vi "Uniform Partially Matched Crossover(UPMX).vi"(9 "indpb":dbl=0.5 format="%#_13g", 10 "Ind 2":T1, 11 "Ind 1":T1) -> (2 "Child 2":T1, 3 "Child 1":T1)   [LabVIEW 2013, in "GA.lvclass"]
uses:
  GA.lvclass
  Controls/Solution_GA.ctl
panel:
  out "Child2 Schedule":u16[](array[numeric])
  out "Child 1 Schedule":u16[](array[numeric])
  out "p2":i32[](array[numeric])
  out "p1":i32[](array[numeric])
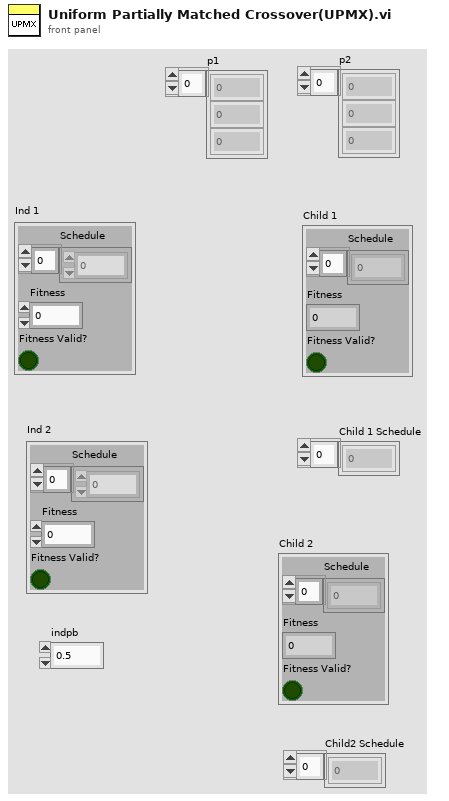
[diagram p1: front panel]
types:
  T1 = typedef "Solution_GA.ctl" = cluster{"Schedule":u16[], "Fitness":u16, "Fitness Valid?":bool}
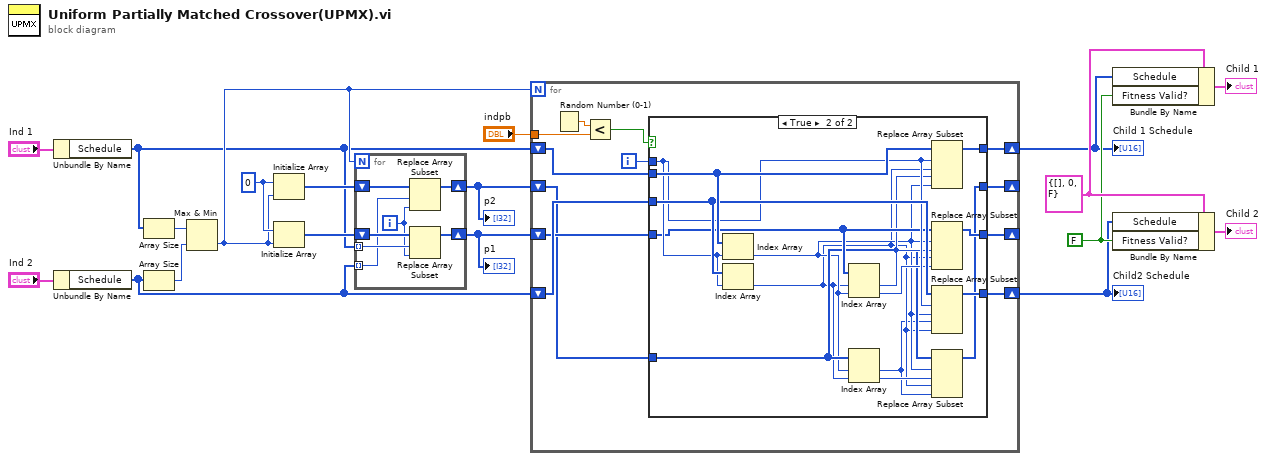
[diagram p0: block diagram]
diagram:
  w9 = FALSE ("Fitness Valid?")
  w10 = T1 {"Schedule"=[], "Fitness"=0, "Fitness Valid?"=FALSE} ("Child 2")
  w17 = 0
  n1 = Unbundle By Name("Ind 1") -> ("Schedule"=w3:u16[])
  n2 = Unbundle By Name("Ind 2") -> ("Schedule"=w1:u16[])
  n3 = Array Size(array=w3) -> (size(s)=w19:i32)
  n4 = Array Size(array=w1) -> (size(s)=w18:i32)
  n5 = Max & Min(x=w19, y=w18) -> (min(x,y)=w14:i32)  [unwired: 1 out]
  n6 = Initialize Array(w17, w14) -> (w15:i32[])
  n7 = Initialize Array(w17, w14) -> (w16:i32[])
  n8 = for {
    N: w14 -> [_]
    tunnel: w3 -> [w24] mode=indexing
    tunnel: w1 -> [w23] mode=indexing
    shift-right: [w21] -> w12
    shift-left: w16 -> [w26]
    shift-right: [w20] -> w11
    shift-left: w15 -> [w25]
    i -> [w22]
    n9 = Replace Array Subset(array=w25, new element=w22, index=w23) -> (w20:i32[])
    n10 = Replace Array Subset(array=w26, new element=w22, index=w24) -> (w21:i32[])
  }
  "p1" <- w12
  "p2" <- w11
  n11 = for {
    N: w14 -> [_]
    tunnel: "indpb" -> [w38]
    shift-right: [w31] -> w6
    shift-left: w3 -> [w36]
    shift-right: [w30] -> w5
    shift-left: w1 -> [w35]
    shift-right: [w29] -> _
    shift-left: w12 -> [w33]
    shift-right: [w28] -> _
    shift-left: w11 -> [w32]
    i -> [w34]
    n12 = Random Number (0-1)() -> (number: 0 to 1=w27:dbl)
    n13 = Less?(x=w27, y=w38) -> (x < y?=w37:bool)
    n14 = case shown="True" w37 {
      tunnel: w36 -> [w42 w57]
      tunnel: w35 -> [w41 w56]
      tunnel: w34 -> [_ w55]
      tunnel: w33 -> [w40 w52]
      tunnel: w32 -> [w39 w48]
      tunnel: [w42 w54] -> w31
      tunnel: [w41 w53] -> w30
      tunnel: [w40 w49] -> w29
      tunnel: [w39 w43] -> w28
      frame False {
      }
      frame True {
        n15 = Index Array(array=w57, index=w55) -> (element=w47:u16)
        n16 = Index Array(array=w56, index=w55) -> (element=w45:u16)
        n17 = Index Array(array=w52, index #1=w45, index #2=w47) -> (element #1=w51:i32, element #2=w50:i32)
        n18 = Index Array(array=w48, index #1=w47, index #2=w45) -> (element #1=w44:i32, element #2=w46:i32)
        n19 = Replace Array Subset(array=w57, new element #1=w45, index #1=w55, new element #2=w47, index #2=w51) -> (w54:u16[])
        n20 = Replace Array Subset(array=w52, new element #1=w51, index #1=w47, new element #2=w50, index #2=w45) -> (w49:i32[])
        n21 = Replace Array Subset(array=w56, new element #1=w47, index #1=w55, new element #2=w45, index #2=w44) -> (w53:u16[])
        n22 = Replace Array Subset(array=w48, new element #1=w46, index #1=w47, new element #2=w44, index #2=w45) -> (w43:i32[])
      }
    }
  }
  "Child 1 Schedule" <- w6
  "Child2 Schedule" <- w5
  n23 = Bundle By Name(cluster=w10, "Schedule"=w6, "Fitness Valid?"=w9) -> (→"Child 1":T1)
  n24 = Bundle By Name(cluster=w10, "Schedule"=w5, "Fitness Valid?"=w9) -> (→"Child 2":T1)
